vi "BodeMagnitudePlot.vi"() -> ()   [LabVIEW 2014]
uses:
  <vilib>/imath/engines/lvmath2/RunTimeEngine/Managers/WorkSpace/UID Generator.vi
  <vilib>/imath/engines/lvmath2/RunTimeEngine/RunTimeType/NIMS_RunTimeType_From StrictType (excl LVString).vi
  <instcachedir>/0/NIMS_RunTimeType_From StrictType (excl LVString)_15A5391EEA9C4AACB9955AC755B83D29.lvgen/NIMS_RunTimeType_From StrictType (excl LVString)_15A5391EEA9C4AACB9955AC755B83D29_000.vi
  <vilib>/imath/engines/lvmath2/RunTimeEngine/LocalVariableDefStatement/MC_LocalVariableDefStatement_Display.vi
  <vilib>/imath/engines/lvmath2/RunTimeEngine/RangeToken/NIMS_Range.vi
  <instcachedir>/0/NIMS_Range_9BCE657718DF4976A877346C61F22738.lvgen/NIMS_Range_9BCE657718DF4976A877346C61F22738_000.vi
  <vilib>/imathl/engines/lvmath/Functions/Error Handling/Create Error.vi
  <vilib>/imath/engines/lvmath2/RunTimeEngine/Managers/SymbolTable/Clear UID.vi
  <vilib>/imath/engines/lvmath2/RunTimeEngine/NodeEndStatement/NIMS_NodeEndStatement_Output.vi
  <instcachedir>/0/NIMS_NodeEndStatement_Output_53EC0D466D134D7ABD903AC30B43404B.lvgen/NIMS_NodeEndStatement_Output_53EC0D466D134D7ABD903AC30B43404B_005.vi
  <vilib>/imath/engines/lvmath2/RunTimeEngine/ErrorHandling/NIMS_Finalize Error.vi
  <vilib>/Analysis/NI_AALPro.lvlib
  <vilib>/imath/engines/lvmath2/RunTimeEngine/Managers/SymbolTable/NIMS_WorkSpace.lvlib
panel:
  in  "Frequency":dbl
  out "XY Graph":cluster{"f":dbl[], "G":dbl[]}[](graph)
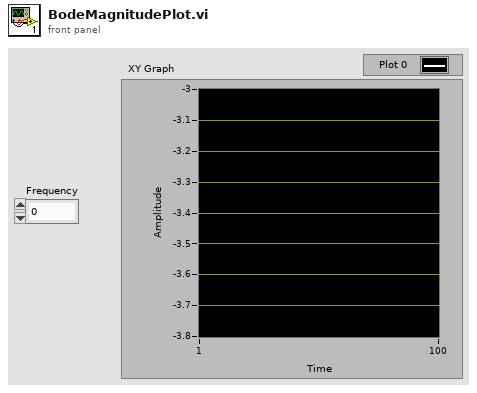
[diagram p1: front panel]
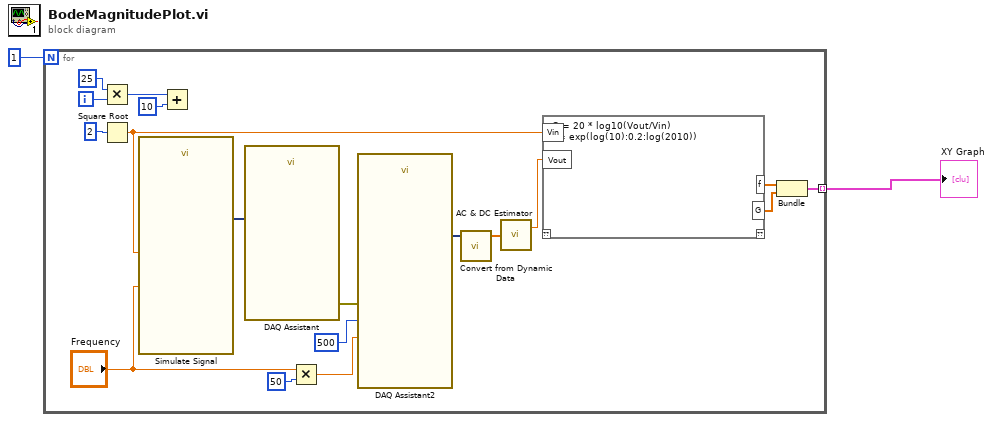
[diagram p0: block diagram]
diagram:
  n1 = for {
    N: 1 -> [_]
    tunnel: [w3] -> w1 mode=indexing
    i -> [w18]
    n2 = Multiply(x=25, y=w18) -> (x*y=w16:i32)
    n3 = Square Root(x=2) -> (sqrt(x)=w8:dbl)
    n4 = call "Simulate Signal"("Frequency"="Frequency", "Amplitude"=w8) -> ("Sine"=w15:dynamicdata)  [unwired: 12 in, 1 out]
    n5 = Add(x=w16, y=10) -> ()  [unwired: 1 out]
    n6 = call "DAQ Assistant"("data"=w15) -> ("error out"=w14:errorcluster)  [unwired: 16 in, 2 out]
    n7 = Multiply(x="Frequency", y=50) -> (x*y=w12:dbl)
    n8 = call "DAQ Assistant2"("rate"=w12, "number of samples"=500, "error in"=w14) -> ("data"=w10:dynamicdata)  [unwired: 14 in, 2 out]
    n9 = call "Convert from Dynamic Data"("Dynamic Data Type"=w10) -> ("Array"=w9:dbl[])  [unwired: 3 in]
    n10 = call <vilib>:"AC & DC Estimator.vi"("Signal (V)"=w9) -> ("AC estimate (Vrms)"=w7:dbl)  [unwired: 1 out]
    n11 = mathscript code="G = 20 * log10(Vout/Vin)\nf = exp(log(10):0.2:log(2010))"("Vin"=w8, "Vout"=w7) -> ("G"=w6:dbl[], "f"=w4:dbl[])  [unwired: 1 in, 1 out]
    n12 = Bundle("f"=w4, "G"=w6) -> (w3:cluster{"f":dbl[], "G":dbl[]})  [unwired: 1 in]
  }
  "XY Graph" <- w1
